vi "Init Database.vi"(8 "error in (no error)":errorcluster, 9 "Database":string, 10 "Resource":string, 11 "Database in":refnum<class "Dummy DB.lvclass">) -> (0 "error out":errorcluster, 3 "Database out":refnum<class "Dummy DB.lvclass">)   [LabVIEW 2020, in "Scratchpad.lvlib" / "Dummy DB.lvclass"]
uses:
  Dummy DB.lvclass
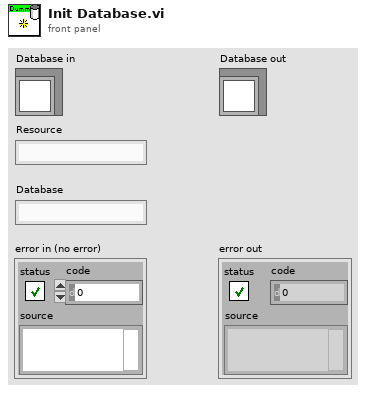
[diagram p1: front panel]
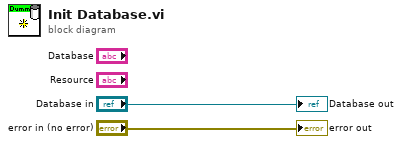
[diagram p0: block diagram]
diagram:
  "error out" <- "error in (no error)"
  "Database out" <- "Database in"
